vi "MapResult Create.vi"(8 "error in (no error)":errorcluster, 10 "InsertResultVariant":variant, 11 "KDBConnection in":refnum<class "DBC.lvclass">) -> (0 "error out":errorcluster, 2 "ID":variant)   [LabVIEW 2020, in "ORM_DBC_Kdb.lvlib" / "DBC.lvclass"]
uses:
  DBC.lvclass
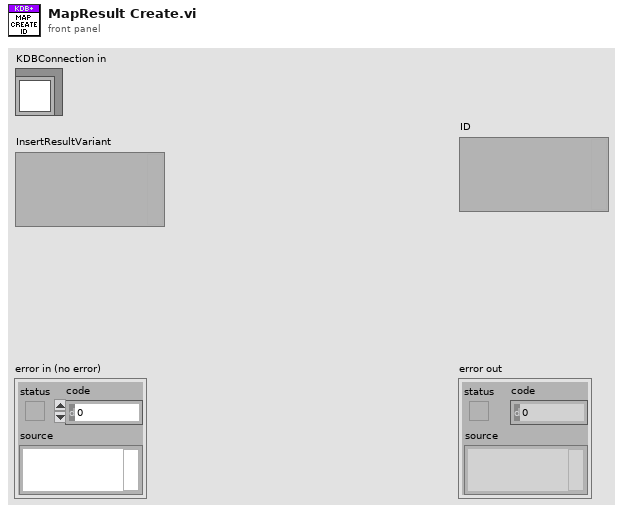
[diagram p1: front panel]
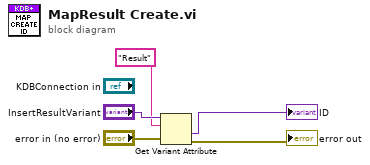
[diagram p0: block diagram]
diagram:
  n1 = Get Variant Attribute(Variant="InsertResultVariant", name="Result", error in="error in (no error)") -> (value=→"ID":variant, error out=→"error out":errorcluster)  [unwired: 1 in, 2 out]
